vi "Serialize Proto.vi"(0 "protoFile ref in":u64, 3 "error in (no error)":errorcluster) -> (7 "protoFile ref out":u64, 8 "outBuffer":string, 10 "error out":errorcluster)   [LabVIEW 2019, in "gRPC Template Creation Utility.lvlib"]
uses:
  gRPC Template Creation Utility.lvlib
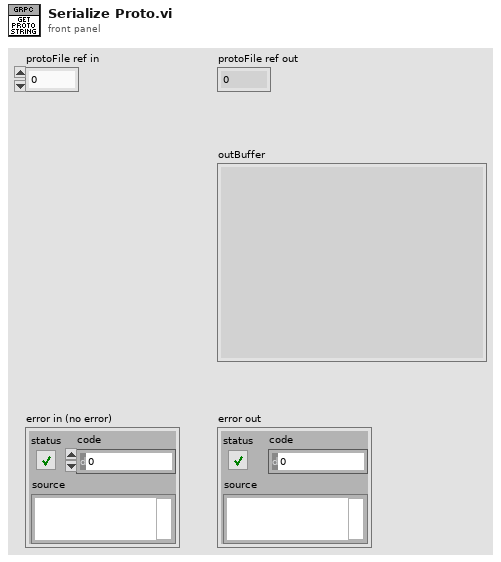
[diagram p1: front panel]
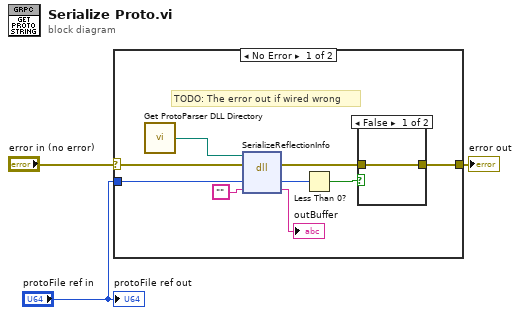
[diagram p0: block diagram]
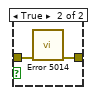
[diagram p2: hidden frame]
diagram:
  n1 = case shown="No Error" "error in (no error)" {
    selector: "error in (no error)" -> [w12 w16]
    tunnel: [w10 w16] -> w2
    tunnel: "protoFile ref in" -> [w8 _]
    frame No Error {
      # "TODO: The error out if wired wrong"
      n2 = call "Get ProtoParser DLL Directory.vi"() -> ("Proto Parser Directory"=w4:path)
      n3 = dll-call lib="?" fn="SerializeReflectionInfo"(path in=w4, error in=w12, "protoRef"=w8, "outBuffer"="") -> (error out=w11:errorcluster, "protoRef"=w6:u64, "outBuffer"=→"outBuffer":string)  [unwired: 2 in, 1 out]
      n4 = Less Than 0?(x=w6) -> (x < 0?=w9:bool)
      n5 = case shown="False" w9 {
        tunnel: w11 -> [w13 w15]
        tunnel: [w13 w14] -> w10
        frame False {
        }
        frame True {
          n6 = call "Error 5014.vi"("error in (no error)"=w15) -> ("error out"=w14:errorcluster)  [unwired: 10 in]
        }
      }
    }
    frame Error {
    }
  }
  "error out" <- w2
  "protoFile ref out" <- "protoFile ref in"
